vi "Emit Message.vi"(8 "error in (no error)":errorcluster, 9 "Priority (Normal)":T1=enum."Normal", 10 "Message":refnum<class "Message.lvclass">, 11 "Actor API in":refnum<class "Actor API.lvclass">) -> (0 "error out":errorcluster, 3 "Actor API out":refnum<class "Actor API.lvclass">)   [LabVIEW 2020, in "Artifex.lvlib" / "Actor API.lvclass"]
uses:
  Actor API.lvclass
  Priority Message Queue/Priority Message Queue.lvclass
  Message/Message.lvclass
  Priority.ctl
  Artifex.lvlib
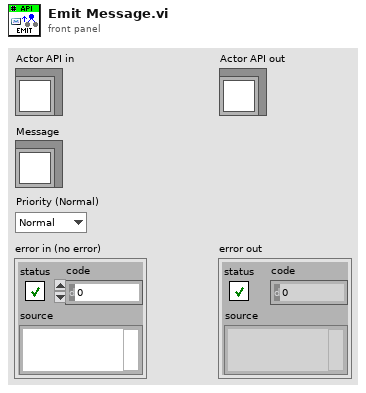
[diagram p1: front panel]
types:
  T1 = typedef "Artifex.lvlib/Priority.ctl" = enum16{"Low", "Normal", "High"}
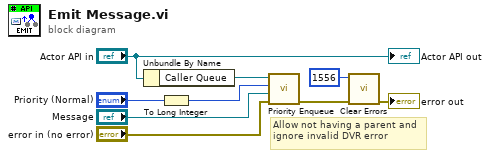
[diagram p0: block diagram]
diagram:
  # "Allow not having a parent and ignore invalid DVR error"
  n1 = Unbundle By Name("Actor API in") -> ("Caller Queue"=w8:refnum<class "Priority Message Queue.lvclass">)
  n2 = To Long Integer(number="Priority (Normal)") -> (32bit integer=w6:i32)
  n3 = call "Priority Enqueue.vi"("error in (no error)"="error in (no error)", "Message"="Message", "Priority"=w6, "Priority Message Queue in"=w8) -> ("error out"=w3:errorcluster)  [unwired: 6 in, 1 out]
  n4 = call <vilib>:"Clear Errors.vi"("error in (no error)"=w3, "specific error code to clear (0: all)"=1556) -> ("error out"=→"error out":errorcluster)  [unwired: 4 in, 1 out]
  "Actor API out" <- "Actor API in"
